vi "getAI.vi"(8 "错误输入（无错误）":errorcluster, 10 "channel":i32, 11 "msg interface":T1) -> (0 "错误输出":errorcluster, 2 "result":dbl format="%#_13g")   [LabVIEW 2013]
panel:
  in  "buff":dbl format="%#_13g"
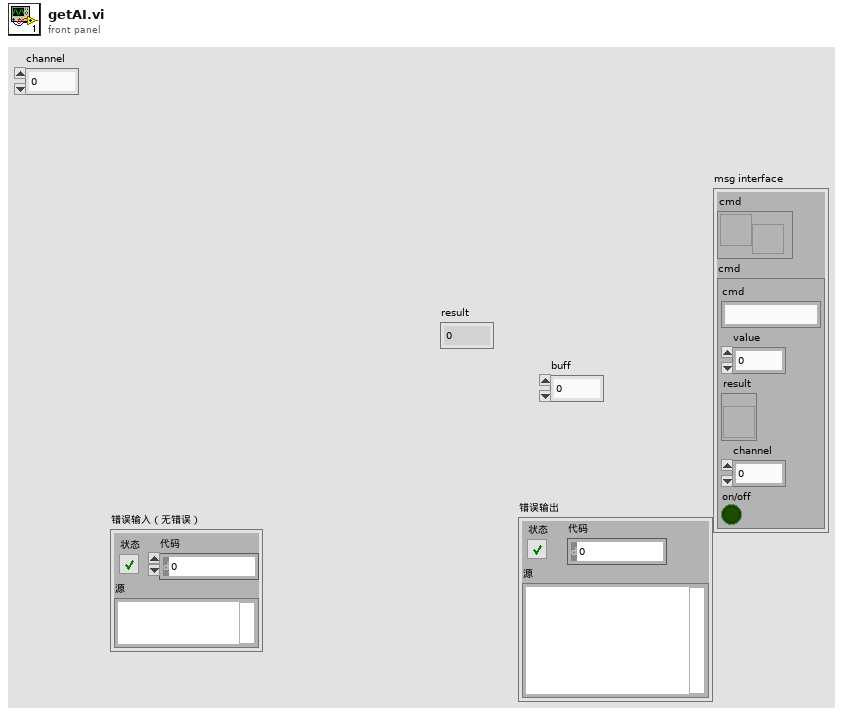
[diagram p1: front panel]
types:
  T1 = cluster{"cmd":refnum<user-event>, "cmd":cluster{"cmd":string, "value":dbl, "result ":refnum<vi>, "channel":i32, "on/off":bool}}
  T2 = cluster{"cmd":string, "value":dbl, "result ":refnum<vi>, "channel":i32, "on/off":bool}
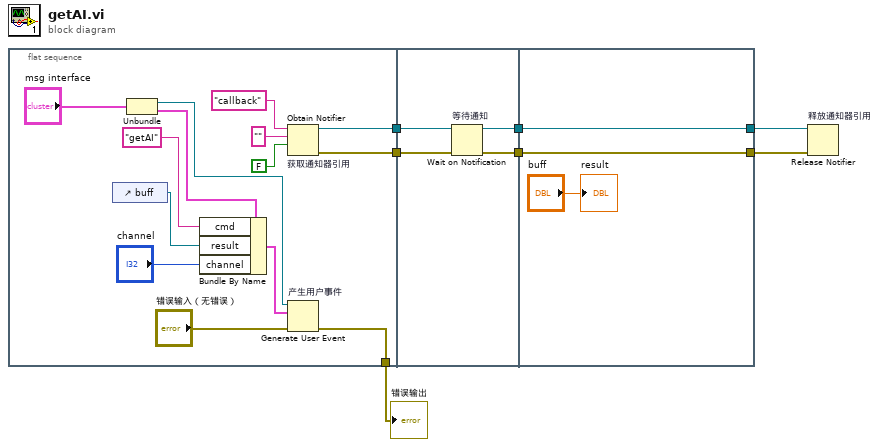
[diagram p0: block diagram]
diagram:
  n1 = flat-sequence {
    tunnel: [w12] -> w7
    tunnel: [w10] -> w6
    tunnel: [w9] -> w5
    tunnel: w7 -> [w25]
    tunnel: w6 -> [w24]
    tunnel: [w23] -> w4
    tunnel: [w22] -> w2
    tunnel: w4 -> [w27]
    tunnel: [w27] -> w3
    tunnel: w2 -> [w26]
    tunnel: [w26] -> w1
    frame #0 {
      n2 = control-ref of="buff"() -> (w21:refnum<vi>)
      n3 = Unbundle("msg interface") -> ("cmd"=w17:refnum<user-event>, "cmd"=w16:T2)
      n4 = Bundle By Name(cluster=w16, "cmd"="getAI", "result"=w21, "channel"="channel") -> (w20:T2)
      n5 = Obtain Notifier "获取通知器引用"(name (unnamed)="callback" ("名称（未命名）"), notification data type="", create if not found? (T)=FALSE ("如未找到是否创建？(T)")) -> (notifier out=w12:refnum<notifier>, error out=w10:errorcluster)  [unwired: 1 in, 1 out]
      n6 = Generate User Event "产生用户事件"(user event=w17, event data cluster=w20, error in="错误输入（无错误）") -> (error out=w9:errorcluster)  [unwired: 1 in, 1 out]
    }
    frame #1 {
      n7 = Wait on Notification "等待通知"(notifier=w25, error in (no error)=w24) -> (notifier out=w23:refnum<notifier>, error out=w22:errorcluster)  [unwired: 2 in, 2 out]
    }
    frame #2 {
      "result" <- "buff"
    }
  }
  n8 = Release Notifier "释放通知器引用"(notifier=w3, error in (no error)=w1) -> ()  [unwired: 1 in, 3 out]
  "错误输出" <- w5
